vi "simple_DFT.vi"(1 "x":dbl[](array[numeric])) -> (0 "X":cdb[](array[numeric]))   [LabVIEW 2013, in "varilib.lvlib"]
doc: "Simple matrix based DFT. Should work with any input sequence size. Returns normalized complex spectrum.\nHowever it is ordinary DFT, not FFT so it will be painfully slow for large sets of 'x'!"
uses:
  varilib.lvlib
  <vilib>/Analysis/baseanly.llb/Real Outer Product.vi
  <vilib>/Analysis/baseanly.llb/Complex A x Vector.vi
  <vilib>/Analysis/Matrix/Numeric/Conversions/Matrix To Array - RM.vi
  <vilib>/Analysis/Matrix/Numeric/Conversions/Array To Matrix - CA2.vi
  <vilib>/Analysis/NI_AALBase.lvlib
  <vilib>/Analysis/Matrix/NI_Matrix.lvlib
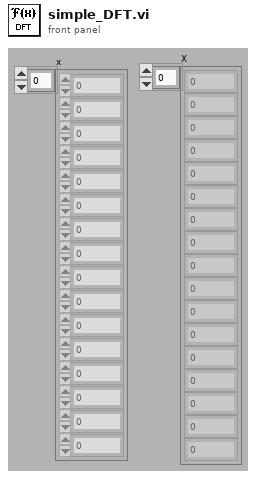
[diagram p1: front panel]
types:
  T1 = typedef "NI_Matrix.lvlib/RealMatrix.ctl" = dbl[][]
  T2 = typedef "NI_Matrix.lvlib/ComplexMatrix.ctl" = cdb[][]
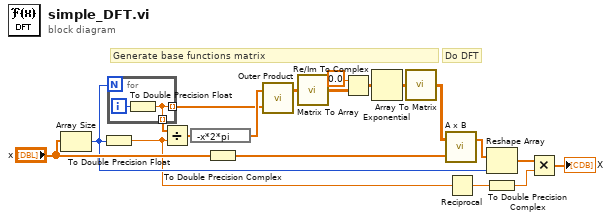
[diagram p0: block diagram]
diagram:
  # "Do DFT"
  # "Generate base functions matrix"
  n1 = Array Size(array="x") -> (size(s)=w17:i32)
  n2 = To Double Precision Float(number=w17) -> (double precision float=w3:dbl)
  n3 = for {
    N: w17 -> [_]
    tunnel: [w20] -> w12 mode=indexing
    tunnel: [w20] -> w15 mode=indexing
    i -> [w21]
    n4 = To Double Precision Float(number=w21) -> (double precision float=w20:dbl)
  }
  n5 = Divide(x=w12, y=w3) -> (x/y=w19:dbl[])
  n6 = expression code="-x*2*pi"(w19) -> (w16:dbl[])
  n7 = To Double Precision Complex(1:"x") -> (0:w14:cdb[])
  n8 = call-poly <vilib>:"Outer Product.vi"("Y Vector"=w15, "X Vector"=w16) -> ("Outer Product"=w10:T1)  [unwired: 1 out]
  n9 = call-poly <vilib>:"Matrix To Array.vi"("Real Matrix"=w10) -> ("Real 2D Array"=w8:dbl[][])
  n10 = Re/Im To Complex ("Cartesian To Complex.vi")(1:w8, 2:0.0 ("Real Scalar r")) -> (0:w11:cdb[][])
  n11 = Exponential ("Exponential.vi")(1:w11) -> (0:w7:cdb[][])
  n12 = call-poly <vilib>:"Array To Matrix.vi"("Complex 2D Array"=w7) -> ("Complex Matrix"=w6:T2)
  n13 = call-poly <vilib>:"A x B.vi"("Vector"=w14, "A"=w6) -> ("A x Vector"=w13:cdb[])  [unwired: 1 out]
  n14 = Reciprocal(x=w3) -> (1/x=w4:dbl)
  n15 = Reshape Array(w13, w17) -> (w5:cdb[])
  n16 = To Double Precision Complex(1:w4) -> (0:w2:cdb)
  n17 = Multiply(x=w5, y=w2) -> (x*y=→"X":cdb[])
